vi "Read xpm.vi"(8 "error in (no error)":errorcluster, 11 "TCSIersStatus in":refnum<class "TCSIersStatus.lvclass">) -> (0 "error out":errorcluster, 2 "xpm":dbl[unit], 3 "TCSIersStatus out":refnum<class "TCSIersStatus.lvclass">)   [LabVIEW 2014, in "TCSDataDefinitions.lvlib" / "TCSTimeComponentStatus.lvlib" / "TCSIersStatus.lvclass"]
uses:
  TCSIersStatus.lvclass
  TCSIersStatus.lvclass/TCSIersStatus.ctl
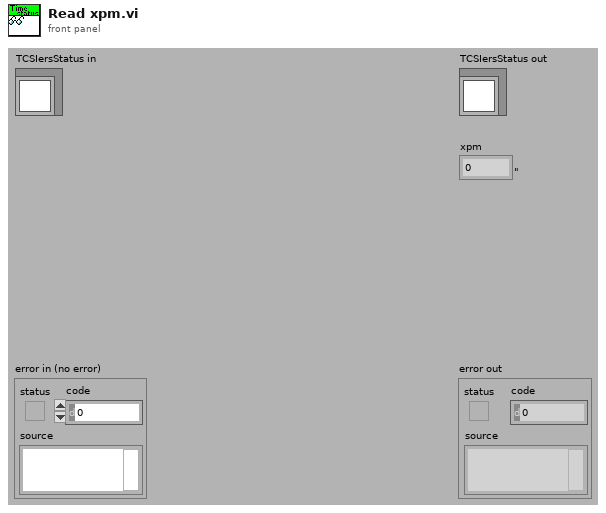
[diagram p1: front panel]
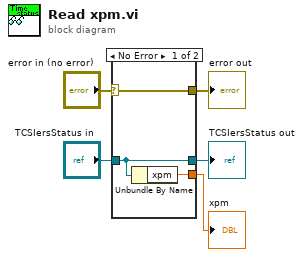
[diagram p0: block diagram]
diagram:
  n1 = case shown="No Error" "error in (no error)" {
    selector: "error in (no error)" -> [w8 w9]
    tunnel: [w8 w9] -> w4
    tunnel: [w7 w10] -> w2
    tunnel: "TCSIersStatus in" -> [w7 w10]
    tunnel: [w6 _] -> w1
    frame No Error {
      n2 = Unbundle By Name(w7) -> ("xpm"=w6:dbl[unit])
    }
    frame Error {
    }
  }
  "error out" <- w4
  "TCSIersStatus out" <- w2
  "xpm" <- w1
